vi "Tester.vi"   [LabVIEW 2019, in "TopModule.lvclass"]
uses:
  Architecture/TopModule/TopModule.lvclass
  Architecture/DMM/DMM.lvclass
  Architecture/ConfigA/ConfigA.lvclass
  Architecture/VoltageMeas/VoltageMeas.lvclass
  C:/Repo/LabVIEW-SOLID-Examples/Architecture/IReference/IReference.lvclass
  C:/Repo/LabVIEW-SOLID-Examples/Architecture/IConfig/IConfig.lvclass
  C:/Repo/LabVIEW-SOLID-Examples/Architecture/IAction/IAction.lvclass
  Architecture/IResult/IResult.lvclass
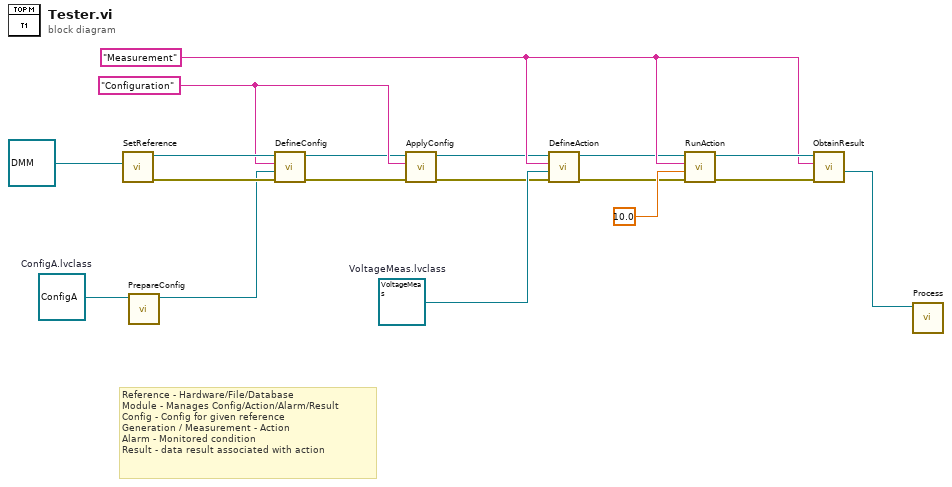
[diagram p0: block diagram]
diagram:
  w16 = refnum<class "VoltageMeas.lvclass"> refnum  # VoltageMeas.lvclass
  w8 = "Measurement" ("Name")
  w10 = refnum<class "ConfigA.lvclass"> refnum  # ConfigA.lvclass
  w15 = "Configuration" ("Name")
  # "Reference - Hardware/File/Database\nModule - Manages Config/Action/Alarm/Result\nConfig - Config for given reference\nGeneration / Measurement - Action\nAlarm - Monitored condition \nResult - data result associated with action"
  n1 = call "SetReference.vi"("Reference"=refnum<class "DMM.lvclass"> refnum ("HWModule.lvclass")) -> ("ErrorOut"=w14:errorcluster, "TopModuleOut"=w17:refnum<class "TopModule.lvclass">)  [unwired: 9 in]
  n2 = call-dynamic "PrepareConfig.vi"("IConfigIn"=w10) -> ("IConfigOut"=w9:refnum<class "ConfigA.lvclass">)  [unwired: 9 in, 1 out]
  n3 = call "DefineConfig.vi"("ErrorIn"=w14, "Config"=w9, "Name"=w15, "TopModuleIn"=w17) -> ("ErrorOut"=w6:errorcluster, "TopModuleOut"=w7:refnum<class "TopModule.lvclass">)  [unwired: 6 in]
  n4 = call "ApplyConfig.vi"("ErrorIn"=w6, "Name"=w15, "TopModuleIn"=w7) -> ("ErrorOut"=w4:errorcluster, "TopModuleOut"=w5:refnum<class "TopModule.lvclass">)  [unwired: 7 in]
  n5 = call "DefineAction.vi"("ErrorIn"=w4, "Measurement"=w16, "Name"=w8, "TopModuleIn"=w5) -> ("ErrorOut"=w2:errorcluster, "TopModuleOut"=w3:refnum<class "TopModule.lvclass">)  [unwired: 6 in]
  n6 = call "RunAction.vi"("ErrorIn"=w2, "Timeout (s)"=10.0, "Action"=w8, "TopModuleIn"=w3) -> ("ErrorOut"=w12:errorcluster, "TopModuleOut"=w13:refnum<class "TopModule.lvclass">)  [unwired: 5 in, 1 out]
  n7 = call "ObtainResult.vi"("ErrorIn"=w12, "Name"=w8, "TopModuleIn"=w13) -> ("ResultOut"=w1:refnum<class "IResult.lvclass">)  [unwired: 5 in, 3 out]
  n8 = call-dynamic "Process.vi"("IResultIn"=w1) -> ()  [unwired: 9 in, 2 out]
